vi "Main.vi"() -> ()   [LabVIEW 2012]
uses:
  <vilib>/Instr/_visa.llb/VISA Flush IO Buffer Mask.ctl
  <vilib>/Instr/_visa.llb/VISA Configure Serial Port (Instr).vi
panel:
  in  "COM Port":refnum<visa-resource-name>="COM5"
  out "Read Buffer":string
  out "Read Buffer (Debug)":string
  out "3D Picture":refnum<vi>(3d-picture)
  out "Elapsed Tme":timestamp format="%<%.3X>T"
  out "return count":u32
  in  "Stop Button":bool
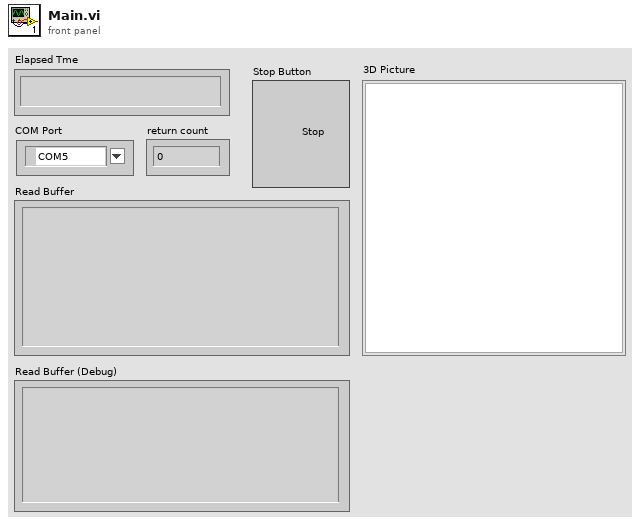
[diagram p1: front panel]
types:
  T1 = typedef "VISA Flush IO Buffer Mask.ctl" = u16
  T2 = enum16{"Raw Acceleration", "Raw Gyro", "Complementy Filter", "Kalman Filter"}
  T3 = cluster{"Numeric Control":dbl, "Numeric Control":dbl, "Numeric Control":dbl}
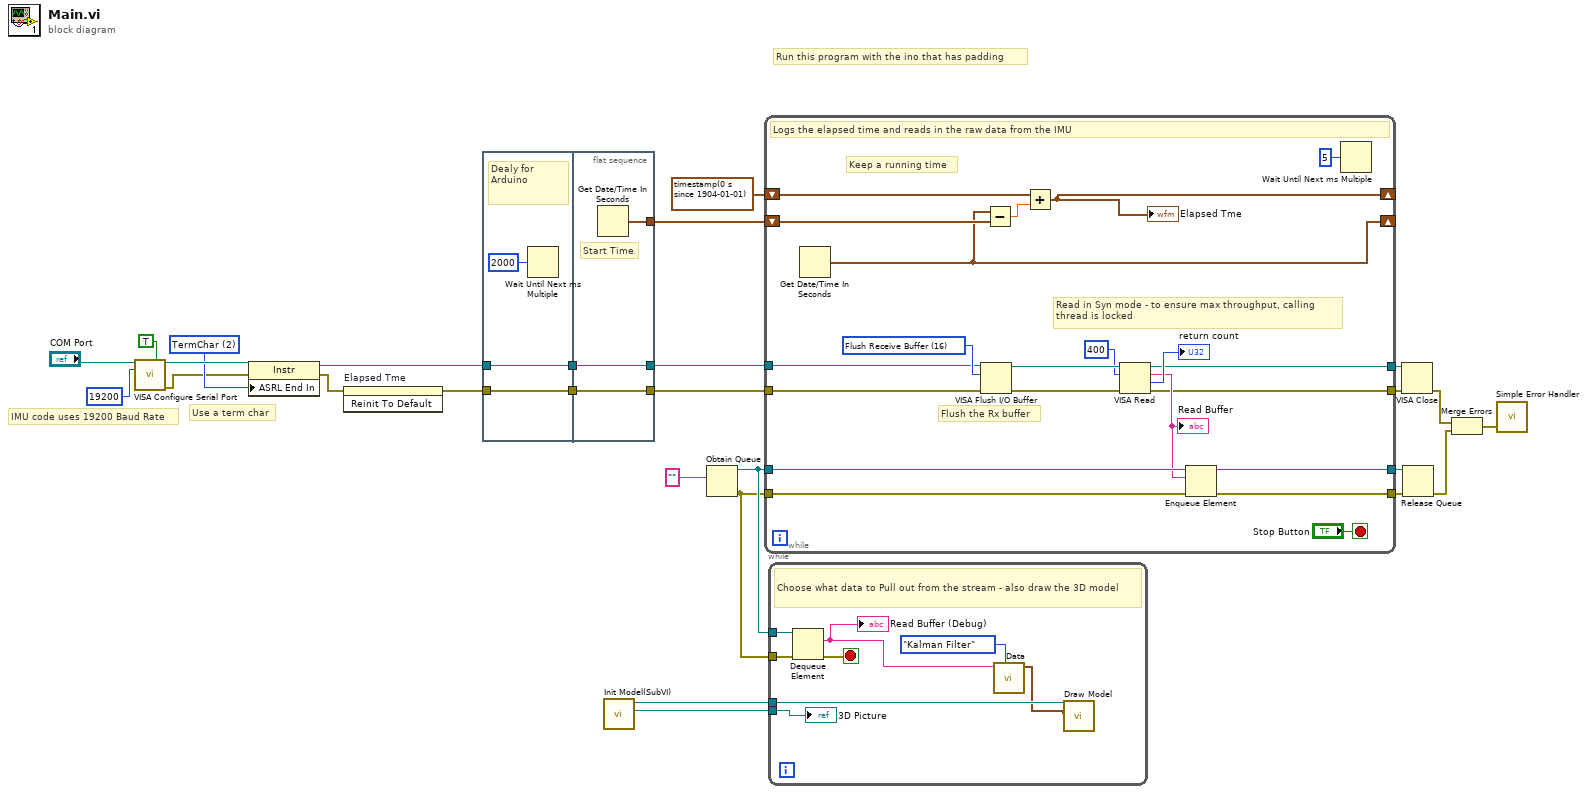
[diagram p0: block diagram]
diagram:
  w20 = u16 2 items=["None", "Last Bit", "TermChar"] ("Serial Settings:End Mode for Reads")
  # "IMU code uses 19200 Baud Rate"
  # "Use a term char"
  # "Run this program with the ino that has padding"
  n1 = call-poly "VISA Configure Serial Port"("VISA resource name"="COM Port", "Enable Termination\nChar (T)"=TRUE ("Enable Termination\nChar (T)"), "baud rate (9600)"=u32 19200) -> ("VISA resource name out"=w21:refnum<visa-resource-name>, "error out"=w19:errorcluster)  [unwired: 11 in]
  n2 = property class="Instr"(reference=w21, error in=w19, "ASRL End In"=w20) -> (reference out=w1:refnum<visa-resource-name>, error out=w3:errorcluster)
  n3 = invoke on="Elapsed Tme" class="AbsTime (strict)" method="Reinit To Default"(error in=w3) -> (error out=w2:errorcluster)  [unwired: 2 in, 2 out]
  n4 = flat-sequence {
    tunnel: w2 -> [w29]
    tunnel: w1 -> [w30]
    tunnel: [w30] -> w5
    tunnel: [w29] -> w4
    tunnel: [w33] -> w8
    tunnel: [w32] -> w7
    tunnel: [w31] -> w6
    tunnel: w5 -> [w33]
    tunnel: w4 -> [w32]
    frame #0 {
      # "Dealy for Arduino"
      n5 = Wait Until Next ms Multiple(millisecond multiple=u32 2000) -> ()  [unwired: 1 out]
    }
    frame #1 {
      # "Start Time"
      n6 = Get Date/Time In Seconds() -> (seconds since 1Jan1904=w31:timestamp)
    }
  }
  n7 = call "Init Model(SubVI).vi"() -> ("Scene:New Object"=w9:refnum<vi>, "SceneObject out"=w10:refnum<vi>)  [unwired: 10 in]
  n8 = Obtain Queue(element data type="") -> (queue out=w23:refnum<queue>, error out=w15:errorcluster)  [unwired: 4 in, 1 out]
  n9 = while {
    tunnel: w8 -> [w39]
    tunnel: w7 -> [w40]
    shift-right: [w43] -> _
    shift-left: w6 -> [w48]
    shift-right: [w44] -> _
    shift-left: timestamp(0 s since 1904-01-01) -> [w47]
    tunnel: w23 -> [w42]
    tunnel: [w41] -> w24
    tunnel: [w37] -> w18
    tunnel: [w36] -> w17
    tunnel: [w35] -> w16
    tunnel: w15 -> [w34]
    stop <- "Stop Button" stop-if-true
    w49 = T1 16 items=["Flush Receive Buffer"=16, "Write Transmit Buffer to Device"=32, "Flush Receive Buffer (No I/O)"=64, "Flush Transmit Buffer"=128] ("Mask")
    # "Read in Syn mode - to ensure max throughput, calling\nthread is locked"
    # "Flush the Rx buffer"
    # "Keep a running time"
    # "Logs the elapsed time and reads in the raw data from the IMU"
    n10 = Get Date/Time In Seconds() -> (seconds since 1Jan1904=w43:timestamp)
    n11 = VISA Flush I/O Buffer(VISA resource name=w39, mask (16)=w49, error in (no error)=w40) -> (VISA resource name out=w52:refnum<visa-resource-name>, error out=w53:errorcluster)
    n12 = Subtract(x=w43, y=w48) -> (x-y=w45:dbl)
    n13 = Add(x=w47, y=w45) -> (x+y=w44:timestamp)
    "Elapsed Tme" <- w44
    n14 = VISA Read(VISA resource name=w52, byte count=u32 400, error in (no error)=w53) -> (VISA resource name out=w37:refnum<visa-resource-name>, read buffer=w38:string, return count=→"return count":u32, error out=w36:errorcluster)
    "Read Buffer" <- w38
    n15 = Enqueue Element(queue=w42, element=w38, error in (no error)=w34) -> (queue out=w41:refnum<queue>, error out=w35:errorcluster)  [unwired: 1 in, 1 out]
    n16 = Wait Until Next ms Multiple(millisecond multiple=u32 5) -> ()  [unwired: 1 out]
  }
  n17 = while {
    tunnel: w23 -> [w62]
    tunnel: w10 -> [w56]
    tunnel: w9 -> [w60]
    tunnel: w15 -> [w58]
    stop <- w61 stop-if-true
    # "Choose what data to Pull out from the stream - also draw the 3D model"
    n18 = Dequeue Element(queue=w62, error in (no error)=w58) -> (element=w59:string, error out=w61:errorcluster)  [unwired: 1 in, 2 out]
    "Read Buffer (Debug)" <- w59
    n19 = call "Data.vi"("Data Type"=T2."Kalman Filter", "Read Buffer"=w59) -> ("XYZ"=w55:T3)  [unwired: 8 in, 1 out]
    n20 = call "Draw Model.vi"("Cluster"=w55, "SceneObject in"=w56) -> ()  [unwired: 9 in, 1 out]
    "3D Picture" <- w60
  }
  n21 = VISA Close(VISA resource name=w18, error in (no error)=w17) -> (error out=w14:errorcluster)
  n22 = Release Queue(queue=w24, error in (no error)=w16) -> (error out=w13:errorcluster)  [unwired: 1 in, 2 out]
  n23 = Merge Errors(w14, w13) -> (w12:errorcluster)
  n24 = call <vilib>:"Simple Error Handler.vi"("error in (no error)"=w12) -> ()  [unwired: 4 in, 5 out]
